vi "Material-SettingsButtonPressed.vi"(8 "error in (no error)":errorcluster, 10 "Boolean":bool, 11 "Cluster in":T1) -> (0 "error out":errorcluster, 3 "Cluster out":T1, 5 "Begin Test Sequence":string)   [LabVIEW 2014, in "Material-RunTest.lvclass"]
uses:
  Material-RunTest.lvclass
  <vilib>/Utility/error.llb/Error Cluster From Error Code.vi
  <vilib>/ErrorRing/Error Ring.xnode
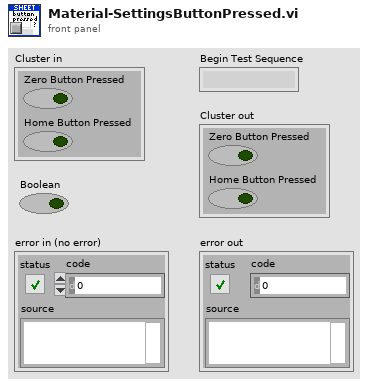
[diagram p1: front panel]
types:
  T1 = cluster{"Zero Button Pressed":bool, "Home Button Pressed":bool}
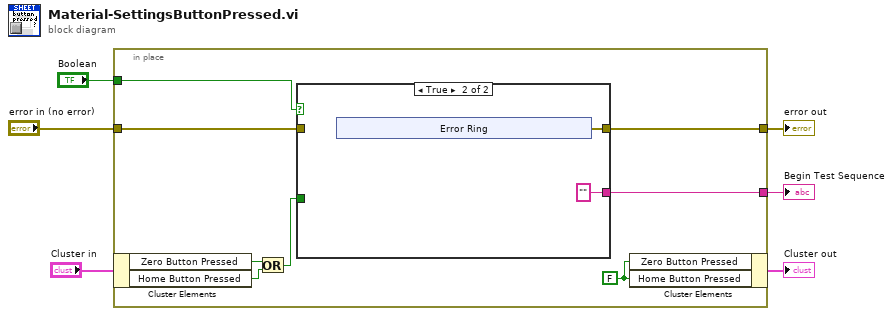
[diagram p0: block diagram]
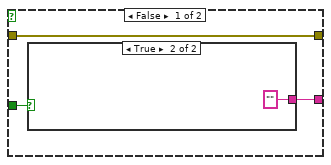
[diagram p2: hidden frame]
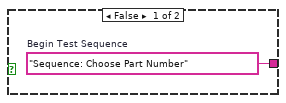
[diagram p3: hidden frame]
diagram:
  n1 = in-place {
    in-place-border: "Boolean" -> [w14]
    in-place-border: [w13] -> w2
    in-place-border: "error in (no error)" -> [w12]
    in-place-border: [w11] -> w4
    w7 = FALSE ("Zero Button Pressed")
    n2 = in-place-cluster #1("Cluster in") -> ("Zero Button Pressed"=w10:bool, "Home Button Pressed"=w9:bool)
    n3 = Or(x=w10, y=w9) -> (x .or. y?=w8:bool)
    n4 = case shown="True" w14 {
      tunnel: [w17 "" ("Begin Test Sequence")] -> w13
      tunnel: w12 -> [w16 _]
      tunnel: [w16 w20] -> w11
      tunnel: w8 -> [w15 _]
      frame False {
        n5 = case shown="True" w15 {
          tunnel: [w18 "" ("Begin Test Sequence")] -> w17
          frame False {
            w18 = "Sequence: Choose Part Number"  # Begin Test Sequence
          }
          frame True {
          }
        }
      }
      frame True {
        n6 = xnode "Error Ring"() -> ("error out"=w20:errorcluster)
      }
    }
    n7 = in-place-cluster #1("Zero Button Pressed"=w7, "Home Button Pressed"=w7) -> (→"Cluster out":T1)
  }
  "error out" <- w4
  "Begin Test Sequence" <- w2
